vi "test.vi"() -> ()   [LabVIEW 2020]
uses:
  <vilib>/Analysis/baseanly.llb/Mean (DBL).vi
  <vilib>/Analysis/NI_AALBase.lvlib
panel:
  out "size(s)":i32
  out "Array":dbl[][](array[numeric])
  out "F-format string":string[](array[string])
  in  "milliseconds to wait":u32
  in  "stop":bool
  in  "Path":path
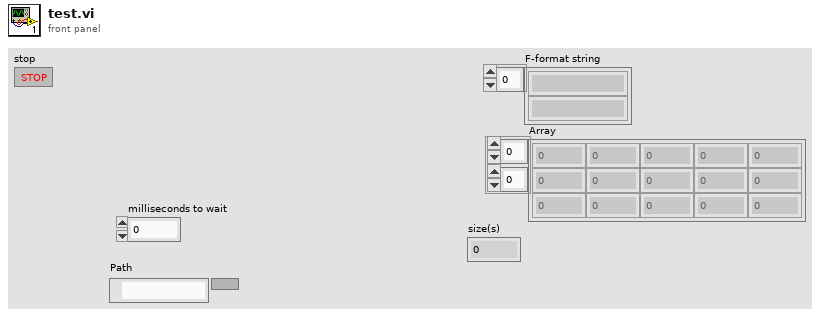
[diagram p1: front panel]
types:
  T1 = enum16{"open", "replace", "create", "open or create", "replace or create", "replace or create with confirmation"}
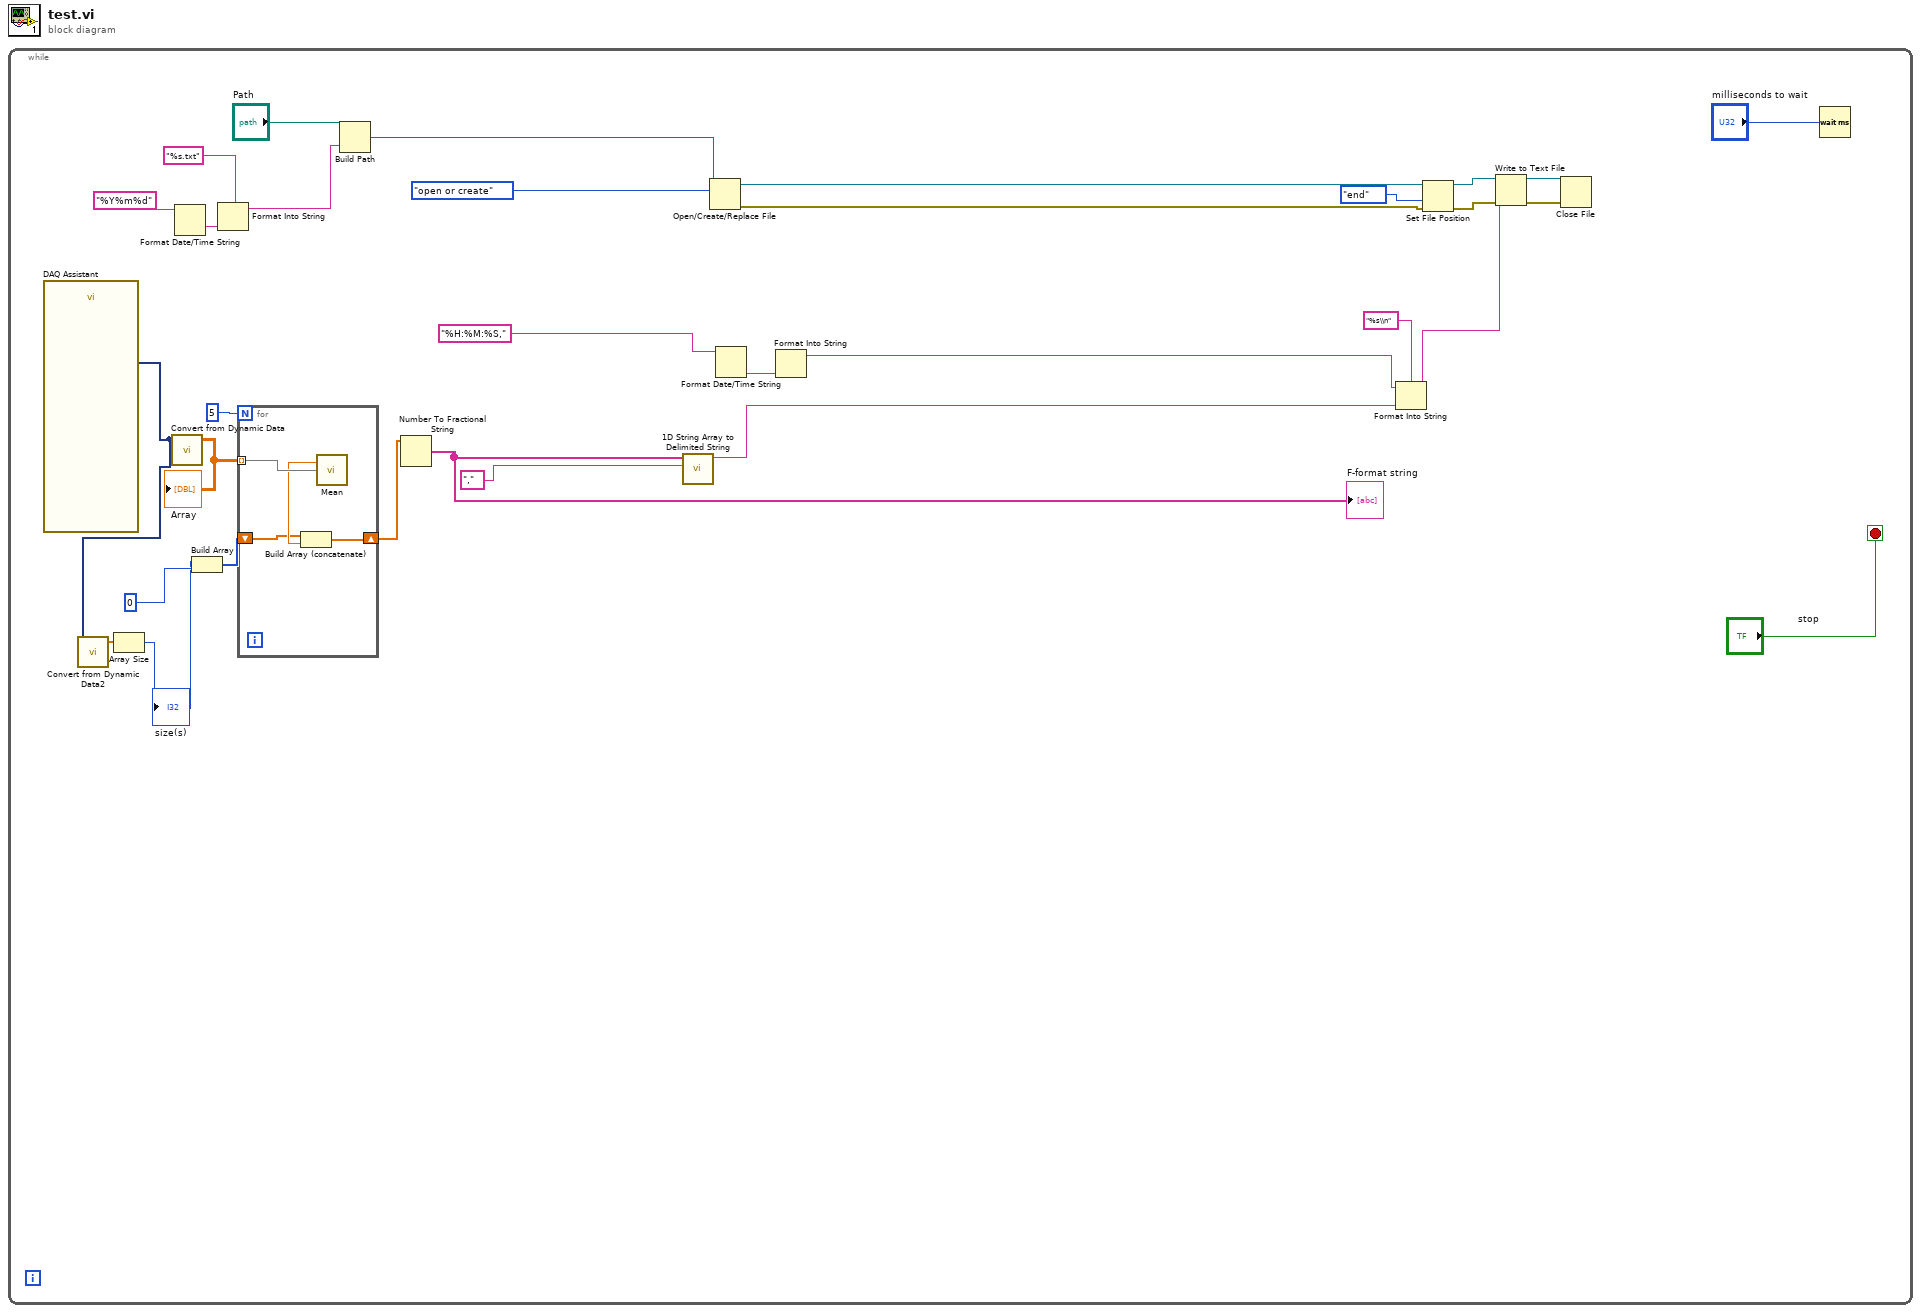
[diagram p0: block diagram]
diagram:
  n1 = while {
    stop <- "stop" stop-if-true
    n2 = call "DAQ Assistant"() -> ("data"=w5:dynamicdata)  [unwired: 16 in, 3 out]
    n3 = call "Convert from Dynamic Data2"("Dynamic Data Type"=w5) -> ("Array"=w4:dbl[])  [unwired: 3 in]
    n4 = Array Size(array=w4) -> (size(s)=w2:i32)
    "size(s)" <- w2
    n5 = call "Convert from Dynamic Data"("Dynamic Data Type"=w5) -> ("Array"=w8:dbl[][])  [unwired: 3 in]
    "Array" <- w8
    n6 = Format Date/Time String(time format string (%c)="%Y%m%d") -> (date/time string=w20:string)  [unwired: 2 in]
    n7 = Build Array(w2, 0 ("element")) -> (w1:i32[])
    n8 = Format Into String(format string="%s.txt", w20) -> (resulting string=w17:string)  [unwired: 2 in, 1 out]
    n9 = for {
      N: 5 -> [_]
      tunnel: w8 -> [w36] mode=indexing
      shift-right: [w34] -> w6
      shift-left: w1 -> [w33]
      n10 = call-poly <vilib>:"Mean.vi"("X"=w36) -> ("mean"=w35:dbl)  [unwired: 1 out]
      n11 = Build Array (concatenate)(w33, w35) -> (w34:dbl[])
    }
    n12 = Build Path(base path="Path", name or relative path=w17) -> (appended path=w16:path)
    n13 = Number To Fractional String(number=w6) -> (F-format string=w9:string[])  [unwired: 3 in]
    "F-format string" <- w9
    n14 = call <vilib>:"1D String Array to Delimited String.vi"("delimiter"="," ("format string"), "string array"=w9) -> ("delimited string"=w15:string)  [unwired: 9 in]
    n15 = Open/Create/Replace File(file path (use dialog)=w16, operation (0:open)=T1."open or create") -> (refnum out=w30:refnum<file>, error out=w27:errorcluster)  [unwired: 4 in, 1 out]
    n16 = Format Date/Time String(time format string (%c)="%H:%M:%S,") -> (date/time string=w11:string)  [unwired: 2 in]
    n17 = Format Into String(w11) -> (resulting string=w10:string)  [unwired: 3 in, 1 out]
    n18 = Format Into String(format string="%s\\n", initial string=w10, w15) -> (resulting string=w22:string)  [unwired: 1 in, 1 out]
    n19 = Set File Position(refnum=w30, from (0:start)=enum16{"start", "end", "current"}."end", error in=w27) -> (refnum out=w29:refnum<file>, error out=w26:errorcluster)  [unwired: 1 in]
    n20 = Write to Text File(file (use dialog)=w29, text=w22, error in=w26) -> (refnum out=w28:refnum<file>, error out=w25:errorcluster)  [unwired: 1 in, 1 out]
    n21 = Close File(refnum=w28, error in=w25) -> ()  [unwired: 2 out]
    n22 = Wait (ms)(milliseconds to wait="milliseconds to wait") -> ()  [unwired: 1 out]
  }
